vi "Untitled 2.vi"(8 "error in (no error)":errorcluster, 11 "Controller in":refnum<class "Controller.lvclass">) -> (0 "error out":errorcluster, 3 "Controller out":refnum<class "Controller.lvclass">)   [LabVIEW 2015, in "Controller.lvclass"]
uses:
  Controller.lvclass
  Controller.lvclass/Controller.ctl
  Mercury Temperature Controller Messages/Set Temperature Msg/Set Temperature Msg.lvclass/Set Temperature Msg.ctl
  <vilib>/ActorFramework/Message Enqueuer/Message Enqueuer.lvclass/Message Enqueuer.ctl
  <vilib>/ActorFramework/Message Enqueuer/Enqueue.vi
  <vilib>/ActorFramework/Message Priority Queue/Priority Enqueue.vi
  Mercury Temperature Controller Messages/Set Temperature Msg/Set Temperature Msg.lvclass
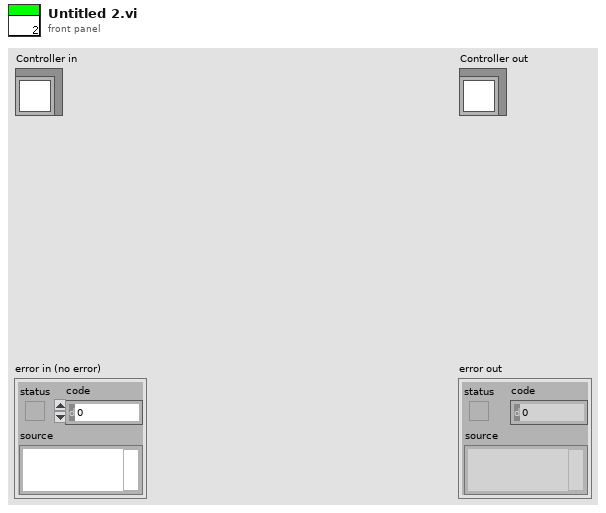
[diagram p1: front panel]
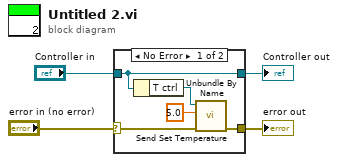
[diagram p0: block diagram]
diagram:
  n1 = case shown="No Error" "error in (no error)" {
    selector: "error in (no error)" -> [w6 w11]
    tunnel: [w5 w11] -> w3
    tunnel: [w9 w10] -> w1
    tunnel: "Controller in" -> [w9 w10]
    frame No Error {
      n2 = Unbundle By Name(w9) -> ("T ctrl"=w8:refnum<class "Message Enqueuer.lvclass">)
      n3 = call "Send Set Temperature.vi"("error in (no error)"=w6, "Temperature setpoint"=5.0, "Message Enqueuer"=w8) -> ("error out"=w5:errorcluster)  [unwired: 7 in, 1 out]
    }
    frame Error {
    }
  }
  "error out" <- w3
  "Controller out" <- w1
